vi "Check Max Number Of Lines.vi"(8 "error in (no error)":errorcluster, 11 "Log in":refnum<class "Log.lvclass">) -> (0 "error out":errorcluster, 3 "Log out":refnum<class "Log.lvclass">)   [LabVIEW 2020, in "Log.lvclass"]
doc: "Test if the number of records written to the file exceeds the specified configuration.\n\nIf it does, then start a new file with the next incremental filename."
uses:
  Log.lvclass
  Log.lvclass/Log.ctl
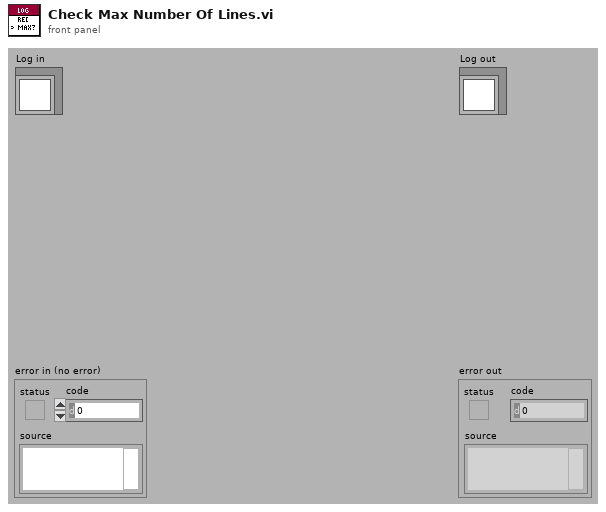
[diagram p1: front panel]
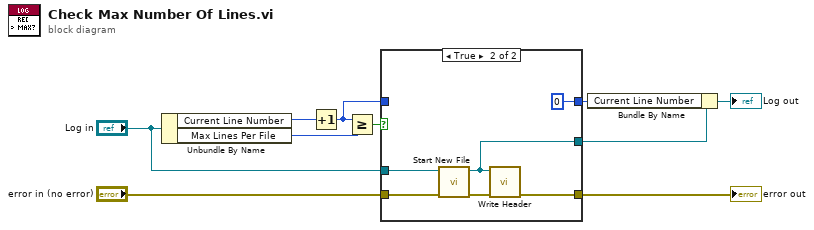
[diagram p0: block diagram]
diagram:
  n1 = Unbundle By Name("Log in") -> ("Current Line Number"=w6:i32, "Max Lines Per File"=w5:i32)
  n2 = Increment(x=w6) -> (x+1=w3:i32)
  n3 = Greater Or Equal?(x=w3, y=w5) -> (x >= y?=w4:bool)
  n4 = case shown="True" w4 {
    tunnel: "Log in" -> [w13 w19]
    tunnel: [w13 w14] -> w1
    tunnel: w3 -> [w12 _]
    tunnel: [w12 0] -> w2
    tunnel: "error in (no error)" -> [w11 w17]
    tunnel: [w11 w15] -> w9
    frame False {
    }
    frame True {
      n5 = call "Start New File.vi"("error in (no error)"=w17, "Log in"=w19) -> ("error out"=w16:errorcluster, "Log out"=w14:refnum<class "Log.lvclass">)  [unwired: 8 out]
      n6 = call "Write Header.vi"("error in (no error)"=w16, "Log in"=w14) -> ("error out"=w15:errorcluster)  [unwired: 1 in, 8 out]
    }
  }
  "error out" <- w9
  n7 = Bundle By Name(cluster=w1, "Current Line Number"=w2) -> (→"Log out":refnum<class "Log.lvclass">)
